vi "CD Config Settings FG.vi"(6 "Action":T2, 7 "UI Refs":T1, 8 "error in (no error)":errorcluster, 10 "CD Settings in":T3={"CD Task Dependency"=18446744073709551615, "CD Task Dependency Ref"=18446744073709551615, "CD Task Available Wfms"=[], "CD Task Selected Wfms"=[], "Buffer Length (s)"=0.0, "Buffer Length (samples)"=0, "Single-point Enabled"=FALSE, "Running Average Enabled"=FALSE, "Task Rate"=0.0} {"CD Task Dependency Ref" format="%.0x"; "CD Task Dependency" format="%.0x"}, 11 "Item Ref":T4 format="%.0x") -> (0 "error out":errorcluster, 2 "CD Settings out":T3={"CD Task Dependency"=18446744073709551615, "CD Task Dependency Ref"=18446744073709551615, "CD Task Available Wfms"=[], "CD Task Selected Wfms"=[], "Buffer Length (s)"=0.0, "Buffer Length (samples)"=0, "Single-point Enabled"=FALSE, "Running Average Enabled"=FALSE, "Task Rate"=0.0} {"CD Task Dependency Ref" format="%.0x"; "CD Task Dependency" format="%.0x"}, 3 "Item Ref out":T4=18446744073709551615 format="%.0x", 5 "UI Refs out":T1)   [LabVIEW 2015, in "Waveform-Processing-Custom-Device Shared.lvlib"]
uses:
  Waveform-Processing-Custom-Device Shared.lvlib
  <vilib>/NI Veristand/Custom Device API/Custom Device Item Ref.ctl
  Custom Device Settings.ctl
  Types/FG Action.ctl
  System Explorer/Types/UI Refs Ctl.ctl
  Constants.vi
  <vilib>/NI Veristand/Custom Device API/Get Item Property (Dependent Node Pointer).vi
  <vilib>/NI Veristand/Custom Device API/Get Item Property (String Array).vi
  <vilib>/NI Veristand/Custom Device API/Get Item Property (Double).vi
  <vilib>/NI Veristand/Custom Device API/Get Item Property (U32).vi
  <vilib>/NI Veristand/Custom Device API/Get Item Property (Boolean).vi
  <vilib>/NI Veristand/Custom Device API/Set Item Property (Dependent Node Pointer).vi
  <vilib>/NI Veristand/Custom Device API/Set Item Property (String Array).vi
  <vilib>/NI Veristand/Custom Device API/Set Item Property (U32).vi
  <vilib>/NI Veristand/Custom Device API/Set Item Property (Boolean).vi
  <vilib>/NI Veristand/Custom Device API/Set Item Property (Double).vi
  <vilib>/NI VeriStand/Custom Device API/Custom Device API.lvlib
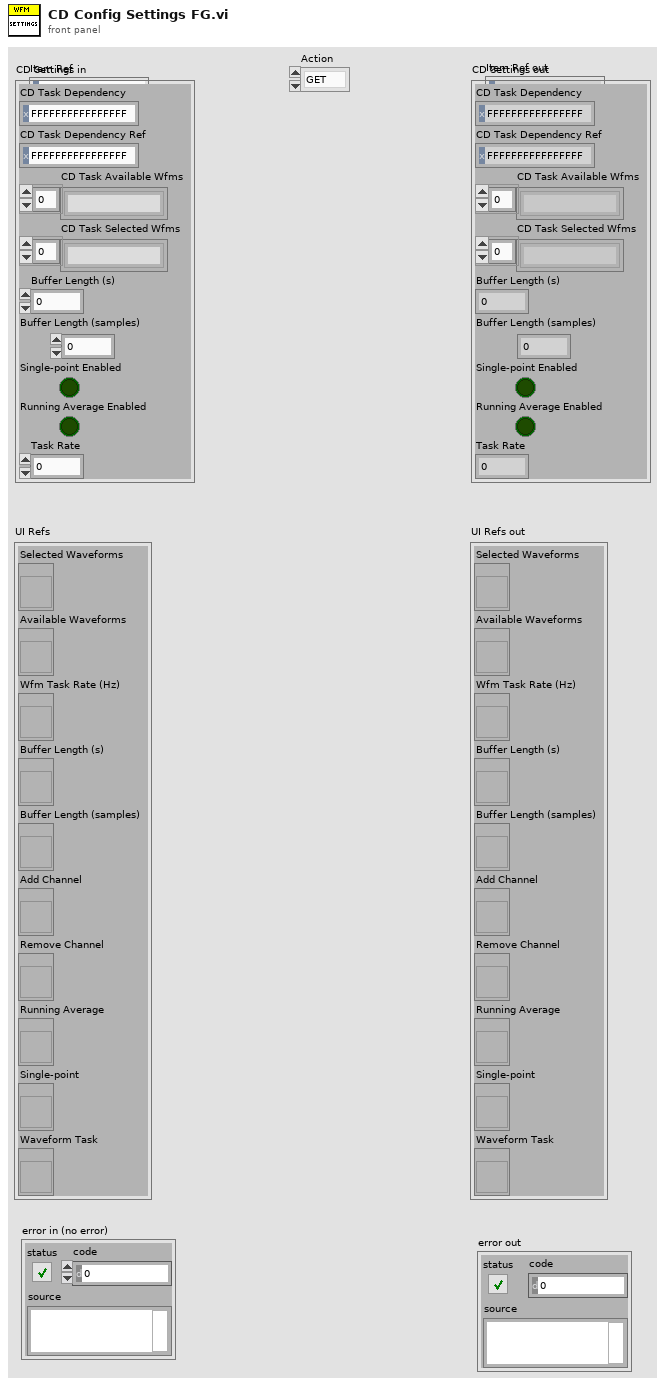
[diagram p1: front panel]
types:
  T1 = typedef "Waveform-Processing-Custom-Device Shared.lvlib/UI Refs Ctl.ctl" = cluster{"Selected Waveforms":refnum<vi>, "Available Waveforms":refnum<vi>, "Wfm Task Rate (Hz)":refnum<vi>, "Buffer Length (s)":refnum<vi>, "Buffer Length (samples)":refnum<vi>, "Add Channel":refnum<vi>, "Remove Channel":refnum<vi>, "Running Average":refnum<vi>, "Single-point":refnum<vi>, "Waveform Task":refnum<vi>}
  T2 = typedef "Waveform-Processing-Custom-Device Shared.lvlib/FG Action.ctl" = enum8{"GET", "SET"}
  T3 = typedef "Waveform-Processing-Custom-Device Shared.lvlib/Custom Device Settings.ctl" = cluster{"CD Task Dependency":T4, "CD Task Dependency Ref":T4, "CD Task Available Wfms":string[], "CD Task Selected Wfms":string[], "Buffer Length (s)":dbl, "Buffer Length (samples)":u32, "Single-point Enabled":bool, "Running Average Enabled":bool, "Task Rate":dbl}
  T4 = typedef "Custom Device API.lvlib/Custom Device Item Ref.ctl" = u64
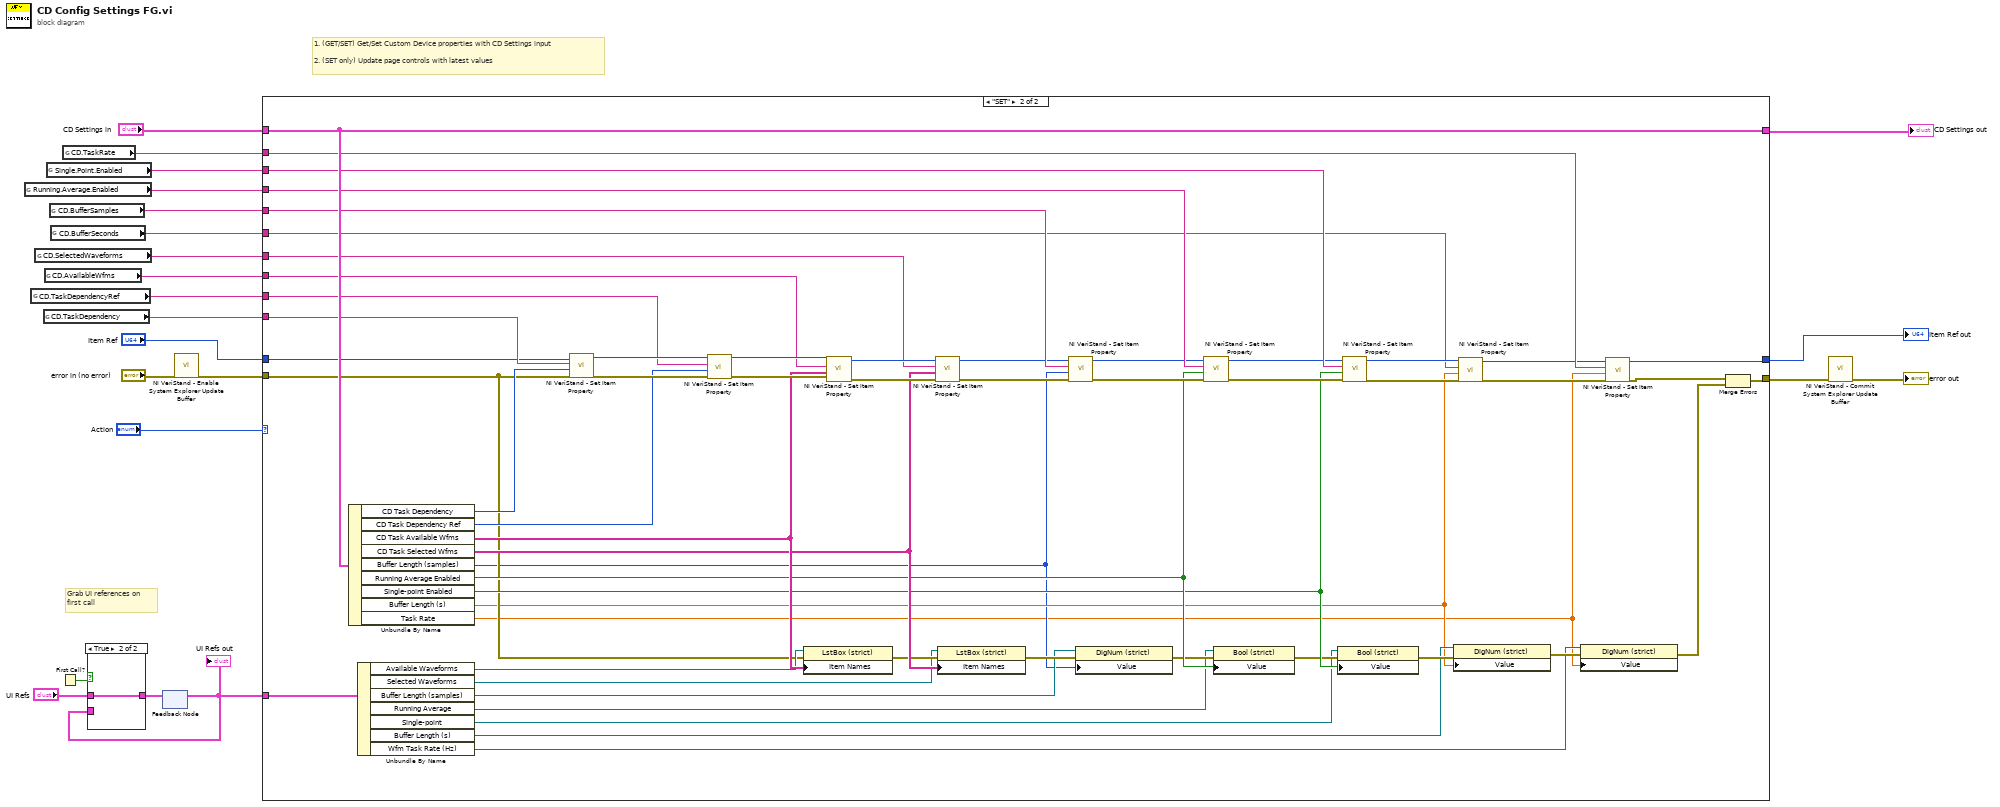
[diagram p0: block diagram]
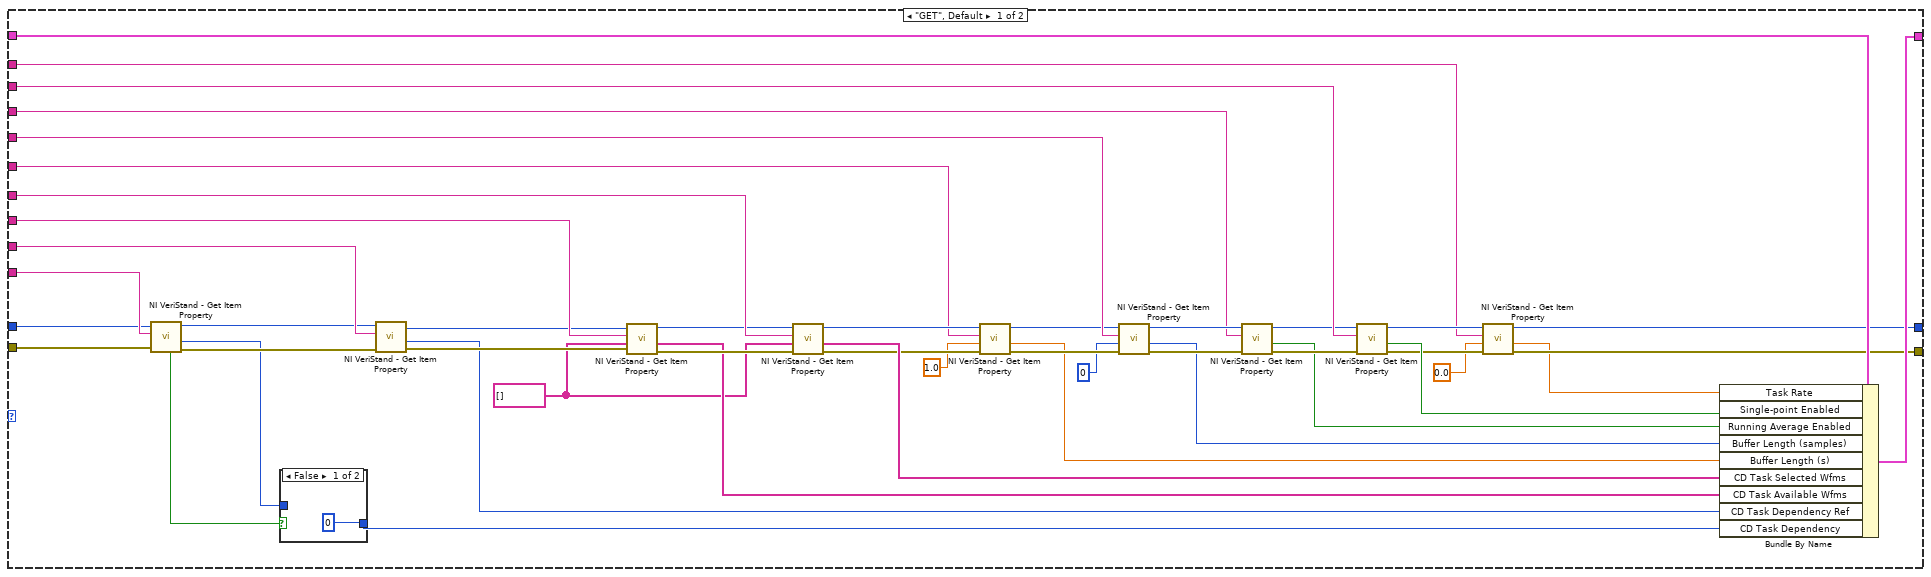
[diagram p3: hidden frame]
diagram:
  # "Grab UI references on\nfirst call"
  # "1. (GET/SET) Get/Set Custom Device properties with CD Settings input\n\n2. (SET only) Update page controls with latest values"
  n1 = global read "Constants.vi" "Running.Average.Enabled"() -> (w18:string)
  n2 = global read "Constants.vi" "CD.TaskDependencyRef"() -> (w21:string)
  n3 = global read "Constants.vi" "CD.SelectedWaveforms"() -> (w19:string)
  n4 = global read "Constants.vi" "CD.TaskDependency"() -> (w22:string)
  n5 = global read "Constants.vi" "CD.AvailableWfms"() -> (w20:string)
  n6 = global read "Constants.vi" "Single.Point.Enabled"() -> (w17:string)
  n7 = global read "Constants.vi" "CD.BufferSamples"() -> (w3:string)
  n8 = global read "Constants.vi" "CD.BufferSeconds"() -> (w2:string)
  n9 = First Call?() -> (First Call?: T/F=w7:bool)
  n10 = global read "Constants.vi" "CD.TaskRate"() -> (w1:string)
  n11 = feedback #1() -> (w4:T1)  [unwired: 1 in]
  "UI Refs out" <- w4
  n12 = case shown="True" w7 {
    tunnel: "UI Refs" -> [_ w24]
    tunnel: [w23 w24] -> w6
    tunnel: w4 -> [w23 _]
    frame False {
    }
    frame True {
    }
  }
  n13 = feedback-in #1(w6) -> ()
  n14 = call <vilib>:"NI VeriStand - Enable System Explorer Update Buffer.vi"("error in (no error)"="error in (no error)") -> ("error out"=w12:errorcluster)  [unwired: 10 in]
  n15 = case shown="\"SET\"" "Action" {
    tunnel: w12 -> [w70 w91]
    tunnel: "Item Ref" -> [w68 w124]
    tunnel: "CD Settings in" -> [w51 w127]
    tunnel: w22 -> [w69 w125]
    tunnel: w21 -> [w66 w122]
    tunnel: w20 -> [w64 w119]
    tunnel: w19 -> [w60 w116]
    tunnel: w3 -> [w58 w114]
    tunnel: w18 -> [w55 w111]
    tunnel: w17 -> [w53 w109]
    tunnel: [w30 w90] -> w9
    tunnel: [w29 w78] -> w10
    tunnel: [w43 w127] -> w16
    tunnel: w4 -> [_ w89]
    tunnel: w2 -> [w35 w84]
    tunnel: w1 -> [w27 w81]
    frame "GET", Default {
      w48 = string[] [] ("Default Value")
      n16 = call-poly <vilib>:"NI VeriStand - Get Item Property.vi"("error in (no error)"=w70, "Property Name"=w69, "Item Ref in"=w68) -> ("error out"=w67:errorcluster, "Dependent Node Ref"=w41:T4, "Item Ref out"=w65:T4, "Found"=w42:bool)  [unwired: 5 in]
      n17 = case shown="False" w42 {
        tunnel: w41 -> [_ w72]
        tunnel: [T4 0 ("Dependent Node Ref") w72] -> w40
        frame False {
        }
        frame True {
        }
      }
      n18 = call-poly <vilib>:"NI VeriStand - Get Item Property.vi"("error in (no error)"=w67, "Property Name"=w66, "Item Ref in"=w65) -> ("error out"=w63:errorcluster, "Dependent Node Ref"=w50:T4, "Item Ref out"=w61:T4)  [unwired: 5 in, 1 out]
      n19 = call-poly <vilib>:"NI VeriStand - Get Item Property.vi"("error in (no error)"=w63, "Default Value"=w48, "Property Name"=w64, "Item Ref in"=w61) -> ("error out"=w62:errorcluster, "Value"=w49:string[], "Item Ref out"=w59:T4)  [unwired: 4 in, 1 out]
      n20 = call-poly <vilib>:"NI VeriStand - Get Item Property.vi"("error in (no error)"=w62, "Default Value"=w48, "Property Name"=w60, "Item Ref in"=w59) -> ("error out"=w39:errorcluster, "Value"=w47:string[], "Item Ref out"=w38:T4)  [unwired: 4 in, 1 out]
      n21 = call-poly <vilib>:"NI VeriStand - Get Item Property.vi"("error in (no error)"=w39, "Default Value"=1.0, "Property Name"=w35, "Item Ref in"=w38) -> ("error out"=w36:errorcluster, "Value"=w33:dbl, "Item Ref out"=w37:T4)  [unwired: 4 in, 1 out]
      n22 = call-poly <vilib>:"NI VeriStand - Get Item Property.vi"("error in (no error)"=w36, "Default Value"=u32 0, "Property Name"=w58, "Item Ref in"=w37) -> ("error out"=w57:errorcluster, "Value"=w46:u32, "Item Ref out"=w56:T4)  [unwired: 4 in, 1 out]
      n23 = call-poly <vilib>:"NI VeriStand - Get Item Property.vi"("error in (no error)"=w57, "Property Name"=w55, "Item Ref in"=w56) -> ("error out"=w54:errorcluster, "Value"=w45:bool, "Item Ref out"=w52:T4)  [unwired: 5 in, 1 out]
      n24 = call-poly <vilib>:"NI VeriStand - Get Item Property.vi"("error in (no error)"=w54, "Property Name"=w53, "Item Ref in"=w52) -> ("error out"=w31:errorcluster, "Value"=w44:bool, "Item Ref out"=w28:T4)  [unwired: 5 in, 1 out]
      n25 = call-poly <vilib>:"NI VeriStand - Get Item Property.vi"("error in (no error)"=w31, "Default Value"=0.0, "Property Name"=w27, "Item Ref in"=w28) -> ("error out"=w30:errorcluster, "Value"=w25:dbl, "Item Ref out"=w29:T4)  [unwired: 4 in, 1 out]
      n26 = Bundle By Name(cluster=w51, "Task Rate"=w25, "Single-point Enabled"=w44, "Running Average Enabled"=w45, "Buffer Length (samples)"=w46, "Buffer Length (s)"=w33, "CD Task Selected Wfms"=w47, "CD Task Available Wfms"=w49, "CD Task Dependency Ref"=w50, "CD Task Dependency"=w40) -> (w43:T3)
    }
    frame "SET" {
      n27 = Unbundle By Name(w127) -> ("CD Task Dependency"=w106:T4, "CD Task Dependency Ref"=w105:T4, "CD Task Available Wfms"=w104:string[], "CD Task Selected Wfms"=w103:string[], "Buffer Length (samples)"=w82:u32, "Running Average Enabled"=w100:bool, "Single-point Enabled"=w98:bool, "Buffer Length (s)"=w83:dbl, "Task Rate"=w74:dbl)
      n28 = Unbundle By Name(w89) -> ("Available Waveforms"=w92:refnum<vi>, "Selected Waveforms"=w93:refnum<vi>, "Buffer Length (samples)"=w94:refnum<vi>, "Running Average"=w95:refnum<vi>, "Single-point"=w96:refnum<vi>, "Buffer Length (s)"=w85:refnum<vi>, "Wfm Task Rate (Hz)"=w75:refnum<vi>)
      n29 = call-poly <vilib>:"NI VeriStand - Set Item Property.vi"("error in (no error)"=w91, "Dependent Node Ref"=w106, "Property Name"=w125, "Item Ref in"=w124) -> ("error out"=w126:errorcluster, "Item Ref out"=w123:T4)  [unwired: 5 in, 1 out]
      n30 = call-poly <vilib>:"NI VeriStand - Set Item Property.vi"("error in (no error)"=w126, "Dependent Node Ref"=w105, "Property Name"=w122, "Item Ref in"=w123) -> ("error out"=w121:errorcluster, "Item Ref out"=w120:T4)  [unwired: 5 in, 1 out]
      n31 = property class="LstBox (strict)"(reference=w92, error in=w91, "Item Names"=w104) -> (error out=w102:errorcluster)  [unwired: 1 out]
      n32 = call-poly <vilib>:"NI VeriStand - Set Item Property.vi"("error in (no error)"=w121, "Value"=w104, "Property Name"=w119, "Item Ref in"=w120) -> ("error out"=w118:errorcluster, "Item Ref out"=w117:T4)  [unwired: 5 in, 1 out]
      n33 = call-poly <vilib>:"NI VeriStand - Set Item Property.vi"("error in (no error)"=w118, "Value"=w103, "Property Name"=w116, "Item Ref in"=w117) -> ("error out"=w115:errorcluster, "Item Ref out"=w113:T4)  [unwired: 5 in, 1 out]
      n34 = property class="LstBox (strict)"(reference=w93, error in=w102, "Item Names"=w103) -> (error out=w101:errorcluster)  [unwired: 1 out]
      n35 = call-poly <vilib>:"NI VeriStand - Set Item Property.vi"("error in (no error)"=w115, "Value"=w82, "Property Name"=w114, "Item Ref in"=w113) -> ("error out"=w112:errorcluster, "Item Ref out"=w108:T4)  [unwired: 5 in, 1 out]
      n36 = property class="DigNum (strict)"(reference=w94, error in=w101, "Value"=w82) -> (error out=w99:errorcluster)  [unwired: 1 out]
      n37 = call-poly <vilib>:"NI VeriStand - Set Item Property.vi"("error in (no error)"=w112, "Value"=w100, "Property Name"=w111, "Item Ref in"=w108) -> ("error out"=w110:errorcluster, "Item Ref out"=w107:T4)  [unwired: 5 in, 1 out]
      n38 = property class="Bool (strict)"(reference=w95, error in=w99, "Value"=w100) -> (error out=w97:errorcluster)  [unwired: 1 out]
      n39 = property class="Bool (strict)"(reference=w96, error in=w97, "Value"=w98) -> (error out=w86:errorcluster)  [unwired: 1 out]
      n40 = call-poly <vilib>:"NI VeriStand - Set Item Property.vi"("error in (no error)"=w110, "Value"=w98, "Property Name"=w109, "Item Ref in"=w107) -> ("error out"=w88:errorcluster, "Item Ref out"=w87:T4)  [unwired: 5 in, 1 out]
      n41 = property class="DigNum (strict)"(reference=w85, error in=w86, "Value"=w83) -> (error out=w76:errorcluster)  [unwired: 1 out]
      n42 = call-poly <vilib>:"NI VeriStand - Set Item Property.vi"("error in (no error)"=w88, "Value"=w83, "Property Name"=w84, "Item Ref in"=w87) -> ("error out"=w80:errorcluster, "Item Ref out"=w77:T4)  [unwired: 5 in, 1 out]
      n43 = property class="DigNum (strict)"(reference=w75, error in=w76, "Value"=w74) -> (error out=w73:errorcluster)  [unwired: 1 out]
      n44 = call-poly <vilib>:"NI VeriStand - Set Item Property.vi"("error in (no error)"=w80, "Value"=w74, "Property Name"=w81, "Item Ref in"=w77) -> ("error out"=w79:errorcluster, "Item Ref out"=w78:T4)  [unwired: 5 in, 1 out]
      n45 = Merge Errors(w79, w73) -> (w90:errorcluster)
    }
  }
  "Item Ref out" <- w10
  "CD Settings out" <- w16
  n46 = call <vilib>:"NI VeriStand - Commit System Explorer Update Buffer.vi"("error in (no error)"=w9) -> ("error out"=→"error out":errorcluster)  [unwired: 10 in]
